vi "SwitcUntilReleased.vi"() -> ()   [LabVIEW 2017]
panel:
  out "NewVal":bool
  in  "stop 2":bool
  out "Numeric":i32
  out "Boolean 2":bool
  in  "Switch until Released":bool
  in  "stop":bool
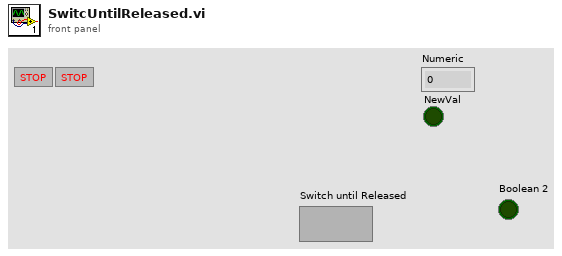
[diagram p1: front panel]
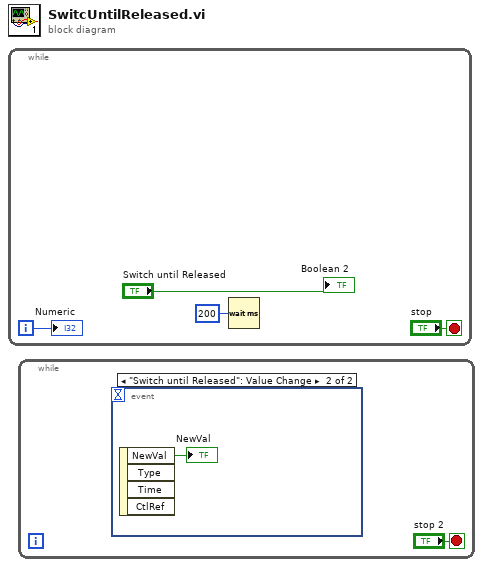
[diagram p0: block diagram]
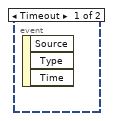
[diagram p2: hidden frame]
diagram:
  n1 = while {
    i -> [w1]
    stop <- "stop" stop-if-true
    n2 = Wait (ms)(milliseconds to wait=u32 200) -> ()  [unwired: 1 out]
    "Boolean 2" <- "Switch until Released"
    "Numeric" <- w1
  }
  n3 = while {
    stop <- "stop 2" stop-if-true
    n4 = event shown="[1] \"Switch until Released\": Value Change" {
      selector: _ -> [_ _]
      dyn-events: _ -> [_ _]
      timeout: _ -> [_ _]
      event Timeout {
        n5 = event-data() -> ()  [unwired: 1 in, 3 out]
      }
      event "Switch until Released": Value Change {
        n6 = event-data() -> ("NewVal"=→"NewVal":bool)  [unwired: 1 in, 3 out]
      }
    }
  }
